vi "input_channel_tester_v2.vi"(10 "Refnums of Controls":T1[](array[typedef])) -> ()   [LabVIEW 2017]
uses:
  <vilib>/gmath/NI_Gmath.lvlib
  <vilib>/Analysis/NI_AALBase.lvlib
  <vilib>/DAQmx/read.llb/DAQmx Read (Analog 1D Wfm NChan NSamp).vi
  <vilib>/Analysis/baseanly.llb/Mean (DBL).vi
  <vilib>/Waveform/WDTOps.llb/WDT Get Waveform Time Array DBL.vi
  <vilib>/DAQmx/configure/timing.llb/DAQmx Timing (Sample Clock).vi
  analog_data.ctl
  Utility Sub VIs/pressure_temp_mixture.ctl
  Utility Sub VIs/pulse_generator_data.ctl
  Utility Sub VIs/pulse_generator_data_charts.ctl
  refnum_array_cluster.ctl
  Utility Sub VIs/diode_charts.ctl
panel:
  in  "Diode ChartsRefnum":refnum<vi>
  in  "PG Charts Refnum":refnum<vi>
  in  "Measurements Data Refnum":refnum<vi>
  in  "Pressure/Temperature/Mixture Properties Refnum":refnum<vi>
  out "Array":T2[](array[typedef])
  out "error out":errorcluster
  in  "stop":bool
  # "Test Section"
  # "Pulse Gen"
  # "Saturation\nPressure [Pa]"
  # "Saturation\nTemperature [C]"
  # "Pressure [Pa]"
  # "Temperature [C]"
  # "Liquid Tank"
  # "Separator"
  # "Liquid Inlet"
  # "Vapor Tank"
  # "Vapor Inlet"
  # "Test Section"
  # "Upper Dev Section"
  # "Lower Dev Section"
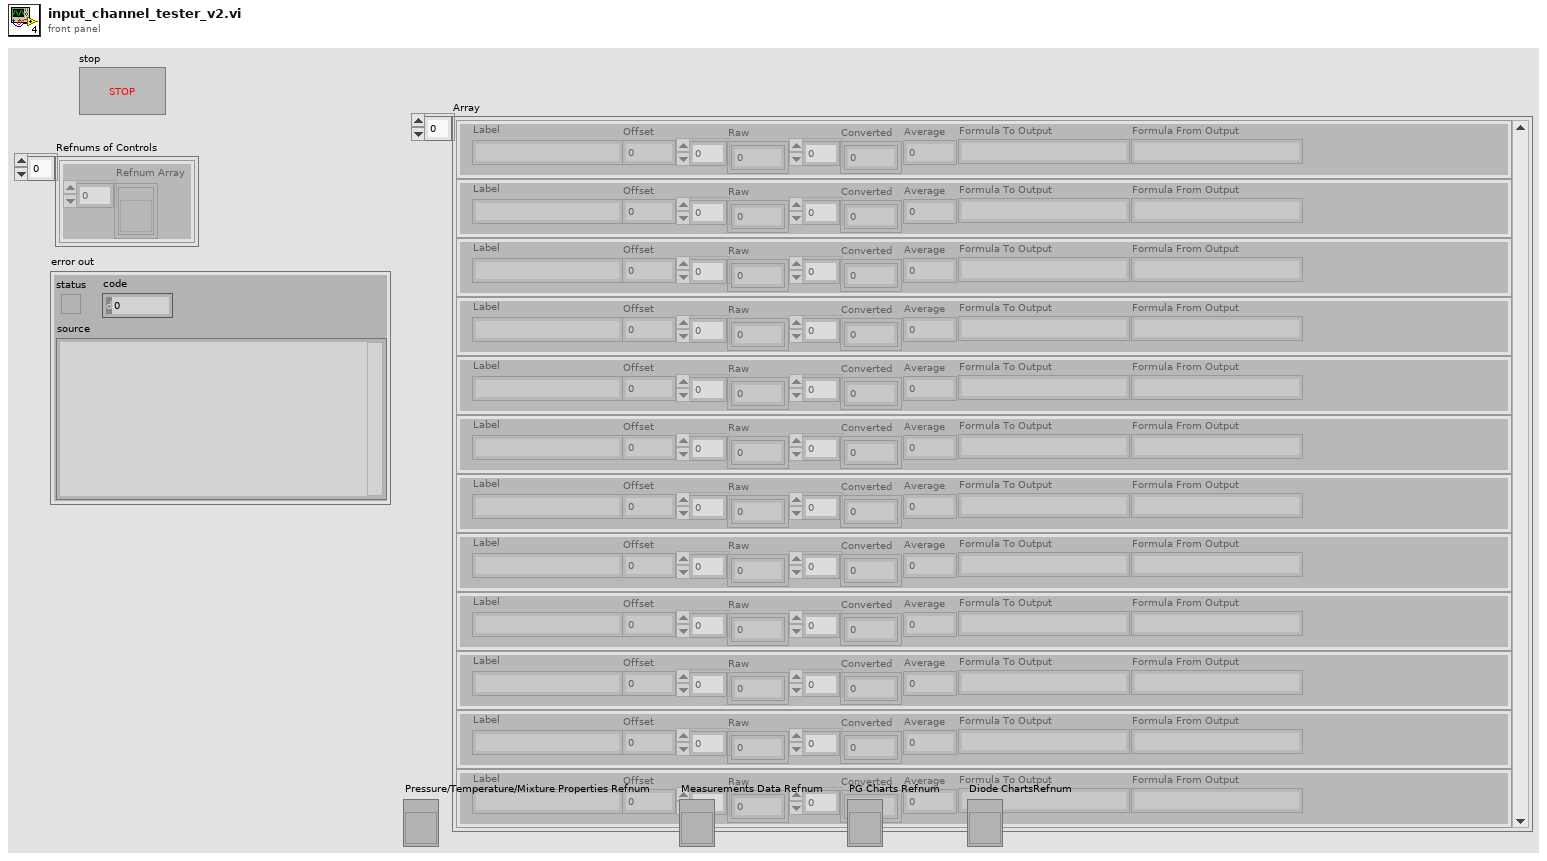
[diagram p1: front panel]
types:
  T1 = typedef "refnum_array_cluster.ctl" = cluster{"Refnum Array":refnum<vi>[]}
  T2 = typedef "analog_data.ctl" = cluster{"Label":string, "Offset":dbl, "Raw":dbl[], "Converted":dbl[], "Average":dbl, "Formula To Output":string, "Formula From Output":string}
  T3 = typedef "analog_data_channel_pkg.ctl" = cluster{"Analog Input Channel":T4, "Analog Data":T2}
  T4 = typedef "input_channel.ctl" = cluster{"Channel Name":string, "Physical Channel":tag, "Sensor Type":enum16{"Absolute Pressure", "Gauge Pressure", "Differential Pressure", "Temperature", "Mass Flow Rate", "Density", "Other"}, "Signal Type":enum16{"Voltage", "Current", "Temperature"}, "Terminal Configuration":i32, "Minimum Value":dbl, "Maximum Value":dbl, "TC Type":i32, "Sensor Min":dbl, "Sensor Max":dbl, "Sensor Offset":dbl, "Sensor Unit":enum16{"psi", "Pa", "inH2O", "inHg", "C", "K", "g/s", "g/cm3", "Volt", "Amp", ""}, "Output Unit":enum16{"psi", "Pa", "inH2O", "inHg", "C", "K", "g/s", "g/cm3", "Volt", "Amp", ""}, "Unit Conversion":dbl, "Active":bool, "Input Type":enum16{"DAQ", "Add-On"}}
  T5 = typedef "index_array_cluster.ctl" = cluster{"Index Array":i32[]}
  T6 = typedef "pressure_temp_mixture.ctl" = cluster{"Line Densities\n[g/cm^3]":cluster{"Vapor Line":dbl, "Liquid Line":dbl}, "Mixture Properties":cluster{"Enthalpy":dbl, "Quality [-]":dbl}, "Component PTs":cluster{"Liquid Tank P":dbl, "Liquid Tank T":dbl, "Liquid Tank Sat P":dbl, "Liquid Tank Sat T":dbl, "Separator P":dbl, "Separator T":dbl, "Separator Sat P":dbl, "Separator Sat T":dbl, "Liquid Inlet P":dbl, "Liquid Inlet T":dbl, "Liquid Inlet Sat P":dbl, "Liquid Inlet Sat T":dbl, "Vapor Tank P":dbl, "Vapor Tank T":dbl, "Vapor Tank Sat P":dbl, "Vapor Tank Sat T":dbl, "Vapor Inlet P":dbl, "Vapor Inlet T":dbl, "Vapor Inlet Sat P":dbl, "Vapor Inlet Sat T":dbl, "Test Section P":dbl, "Test Section T":dbl, "Test Section Sat P":dbl, "Test Section Sat T":dbl, "Upper Dev Section P":dbl, "Upper Dev Section T":dbl, "Upper Dev Section Sat P":dbl, "Upper Dev Section Sat T":dbl, "Lower Dev Section P":dbl, "Lower Dev Section T":dbl, "Lower Dev Section Sat P":dbl, "Lower Dev Section Sat T":dbl}, "Ambient Pressure [Pa]":dbl, "Mixing Tee":cluster{"Venturi dP":dbl, "PGminiPressure":dbl, "PGminiTemperature":dbl}}
  T7 = cluster{"[0]":dbl, "[1]":dbl, "[2]":dbl, "[3]":dbl, "[4]":dbl, "[5]":dbl, "[6]":dbl, "[7]":dbl, "[8]":dbl, "[9]":dbl, "[10]":dbl, "[11]":dbl, "[12]":dbl, "[13]":dbl, "[14]":dbl, "[15]":dbl, "[16]":dbl, "[17]":dbl, "[18]":dbl, "[19]":dbl, "[20]":dbl, "[21]":dbl, "[22]":dbl, "[23]":dbl, "[24]":dbl, "[25]":dbl, "[26]":dbl, "[27]":dbl, "[28]":dbl, "[29]":dbl, "[30]":dbl, "[31]":dbl}
  T8 = cluster{"Mass Flow Rate [g/s]":dbl, "Mass Flow Rate [g/s]":dbl}
  T9 = cluster{"[0]":dbl, "[1]":dbl, "[2]":dbl, "[3]":dbl, "[4]":dbl, "[5]":dbl, "[6]":dbl, "[7]":dbl, "[8]":dbl, "[9]":dbl, "[10]":dbl, "[11]":dbl, "[12]":dbl, "[13]":dbl, "[14]":dbl, "[15]":dbl}
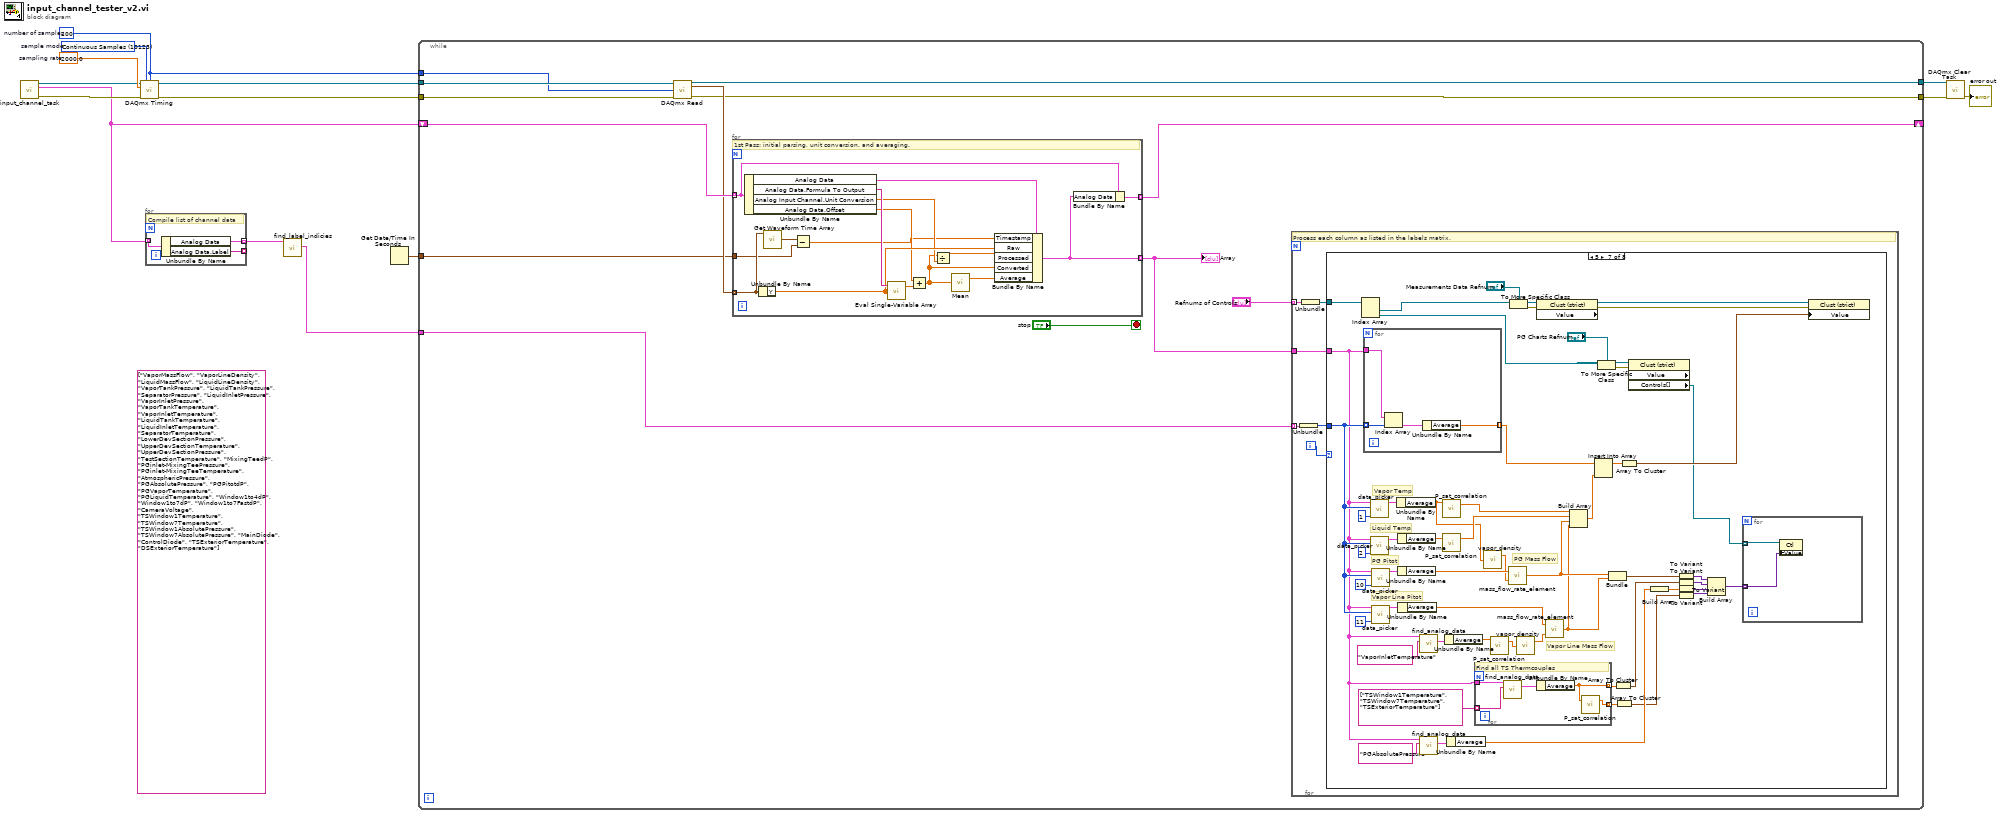
[diagram p0: block diagram]
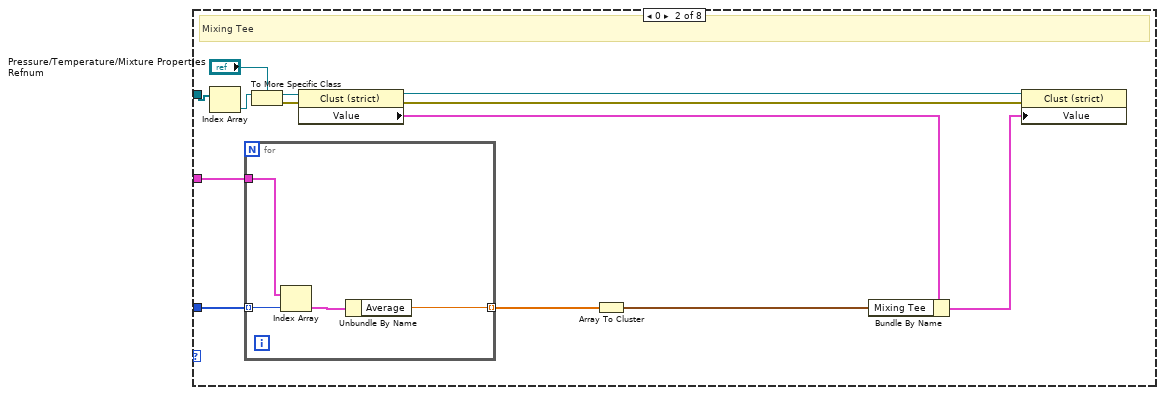
[diagram p3: hidden frame]
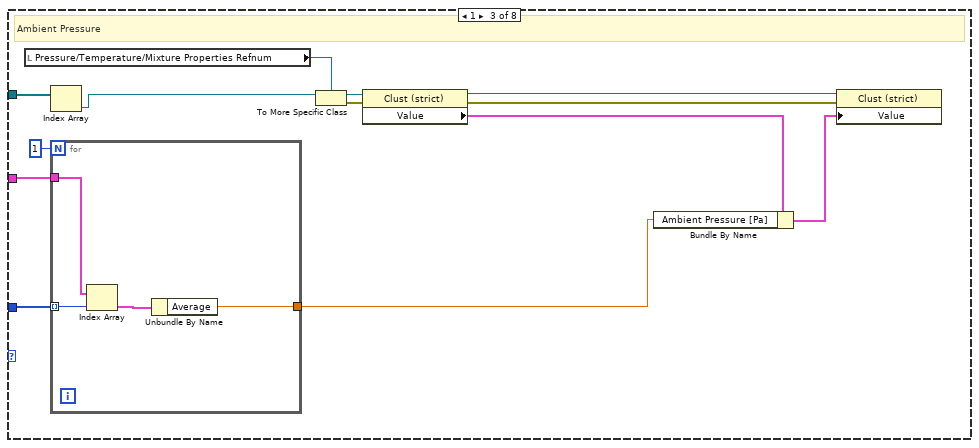
[diagram p4: hidden frame]
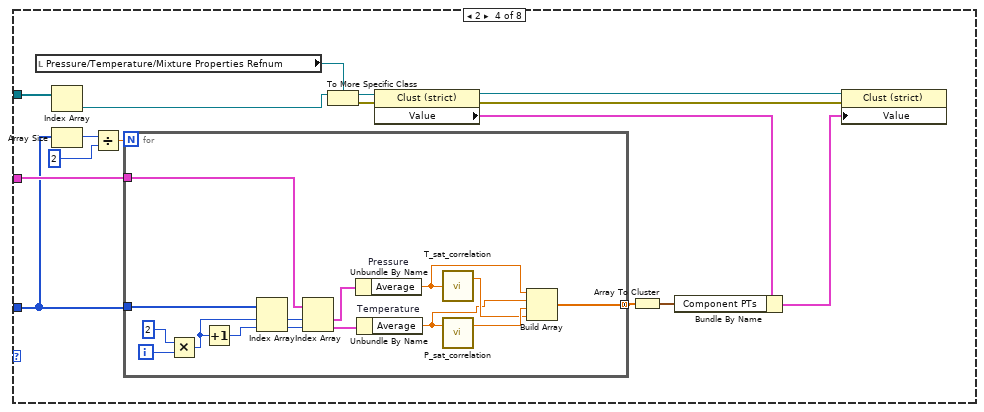
[diagram p5: hidden frame]
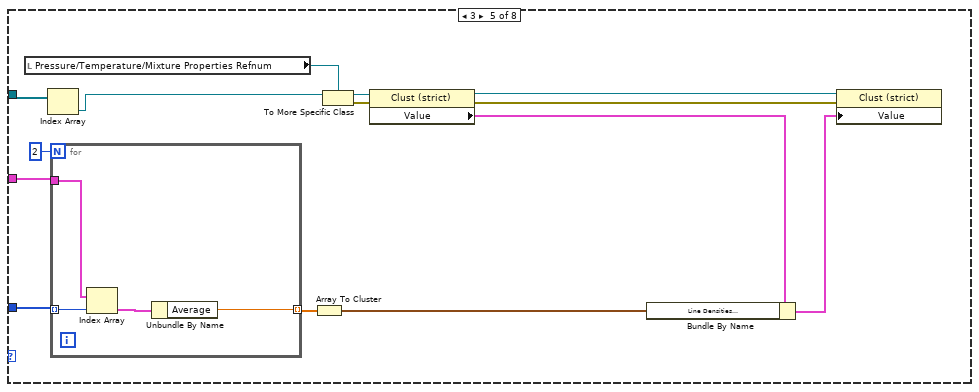
[diagram p6: hidden frame]
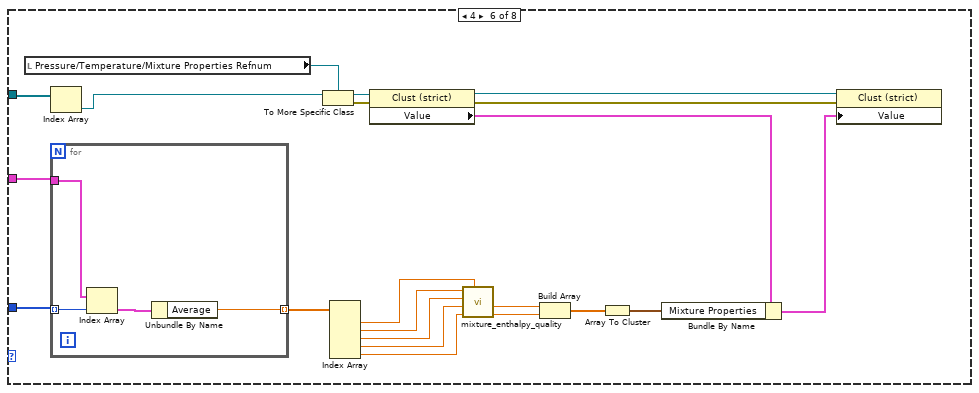
[diagram p7: hidden frame]
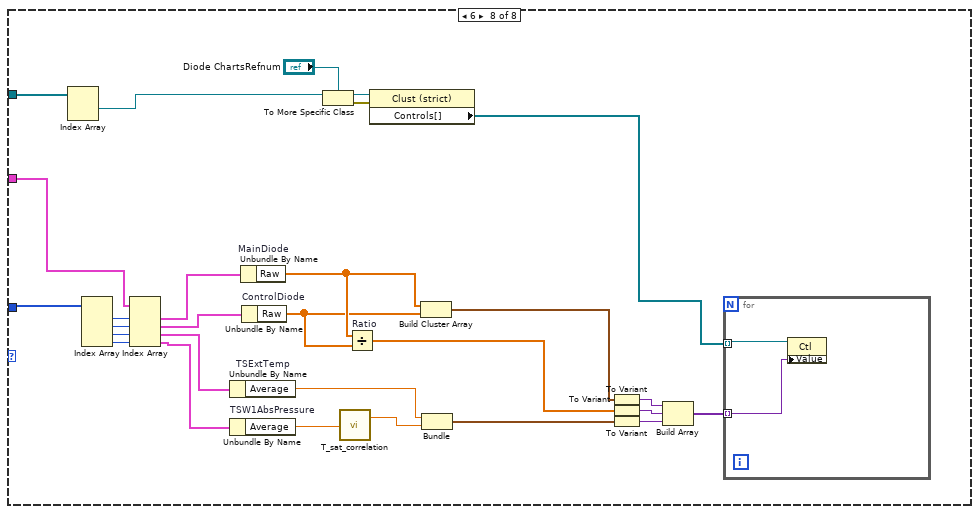
[diagram p8: hidden frame]
diagram:
  (unwired) string[] ["VaporMassFlow", "VaporLineDensity", "LiquidMassFlow", "LiquidLineDensity", "VaporTankPressure", "LiquidTankPressure", "SeparatorPressure", "LiquidInletPressure", "VaporInletPressure", "VaporTankTemperature", "VaporInletTemperature", "LiquidTankTemperature", "LiquidInletTemperature", "SeparatorTemperature", "LowerDevSectionPressure", "UpperDevSectionTemperature", "UpperDevSectionPressure", "TestSectionTemperature", "MixingTeedP", "PGinlet-MixingTeePressure", "PGinlet-MixingTeeTemperature", "AtmosphericPressure", "PGAbsolutePressure", "PGPitotdP", "PGVaporTemperature", "PGLiquidTemperature", "Window1to4dP", "Window1to7dP", "Window1to7FastdP", "CameraVoltage", "TSWindow1Temperature", "TSWindow7Temperature", "TSWindow1AbsolutePressure", "TSWindow7AbsolutePressure", "MainDiode", "ControlDiode", "TSExteriorTemperature", "DSExteriorTemperature"] ("Array 2")
  w14 = 10123 items=["Finite Samples"=10178, "Continuous Samples"=10123, "Hardware Timed Single Point"=12522]  # sample mode
  w13 = 2000.0  # sampling rate
  w4 = 200  # number of samples
  n1 = call "input_channel_task.vi"() -> ("error out"=w11:errorcluster, "Active Analog Channel-Data Packages"=w3:T3[], "task out"=w12:refnum<k21>)  [unwired: 9 in]
  n2 = call-poly <vilib>:"DAQmx Timing.vi"("task/channels in"=w12, "sample mode"=w14, "samples per channel"=w4, "rate"=w13, "error in"=w11) -> ("task out"=w10:refnum<k21>, "error out"=w9:errorcluster)  [unwired: 9 in]
  n3 = for {
    tunnel: w3 -> [w17] mode=indexing
    tunnel: [w16] -> w2 mode=indexing
    tunnel: [w15] -> _ mode=indexing
    # "Compile list of channel data"
    n4 = Unbundle By Name(w17) -> ("Analog Data"=w16:T2, "Analog Data.Label"=w15:string)
  }
  n5 = call "find_label_indicies.vi"("haystack"=w2) -> ("Indicies"=w1:T5[])  [unwired: 8 in, 2 out]
  n6 = Get Date/Time In Seconds() -> (seconds since 1Jan1904=w5:timestamp)
  n7 = while {
    tunnel: w10 -> [w28]
    tunnel: w9 -> [w27]
    tunnel: [w25] -> w7
    tunnel: [w24] -> w8
    tunnel: w5 -> [w23]
    tunnel: w4 -> [w22]
    tunnel: w1 -> [w19]
    shift-right: [w20] -> _
    shift-left: w3 -> [w29]
    stop <- "stop" stop-if-true
    n8 = call-poly <vilib>:"DAQmx Read.vi"("task/channels in"=w28, "number of samples per channel"=w22, "error in"=w27) -> ("task out"=w24:refnum<k21>, "data"=w26:waveform(dbl)[], "error out"=w25:errorcluster)  [unwired: 10 in]
    n9 = for {
      tunnel: w29 -> [w243] mode=indexing
      tunnel: w26 -> [w255] mode=indexing
      tunnel: [w242] -> w21 mode=indexing
      tunnel: w23 -> [w245]
      tunnel: [w241] -> w20 mode=indexing
      # "1st Pass: initial parsing, unit conversion, and averaging."
      n10 = Unbundle By Name(w243) -> ("Analog Data"=w256:T2, "Analog Data.Formula To Output"=w254:string, "Analog Input Channel.Unit Conversion"=w251:dbl, "Analog Data.Offset"=w247:dbl)
      n11 = Unbundle By Name(w255) -> ("Y"=w253:dbl[])
      n12 = call-poly <vilib>:"Get Waveform Time Array.vi"("waveform in"=w255) -> ("X array"=w246:timestamp[])  [unwired: 9 in, 1 out]
      n13 = Subtract(x=w246, y=w245) -> (x-y=w244:dbl[])
      n14 = call <vilib>:"Eval Single-Variable Array.vi"("X Values"=w253, "formula"=w254) -> ("Y Values"=w249:dbl[])  [unwired: 1 in, 1 out]
      n15 = Add(x=w247, y=w249) -> (x+y=w248:dbl[])
      n16 = Divide(x=w248, y=w251) -> (x/y=w250:dbl[])
      n17 = call-poly <vilib>:"Mean.vi"("X"=w248) -> ("mean"=w252:dbl)  [unwired: 1 out]
      n18 = Bundle By Name(cluster=w256, "Timestamp"=w244, "Raw"=w253, "Processed"=w250, "Converted"=w248, "Average"=w252) -> (w242:T2)
      n19 = Bundle By Name(cluster=w243, "Analog Data"=w242) -> (w241:T3)
    }
    "Array" <- w21
    n20 = for {
      tunnel: w21 -> [w35]
      tunnel: w19 -> [w32] mode=indexing
      tunnel: "Refnums of Controls" -> [w34] mode=indexing
      i -> [w36]
      # "Process each column as listed in the labels matrix."
      n21 = Unbundle(w32) -> ("Index Array"=w31:i32[])
      n22 = Unbundle(w34) -> ("Refnum Array"=w33:refnum<vi>[])
      n23 = case shown="5" w36 {
        tunnel: w31 -> [_ w42 w59 w78 w107 w132 w186 w228]
        tunnel: w33 -> [_ w38 w55 w72 w103 w121 w156 w234]
        tunnel: w35 -> [_ w41 w60 w79 w108 w133 w161 w226]
        frame Default {
        }
        frame 0 {
          # "Mixing Tee"
          n24 = Index Array(array=w38) -> (element=w37:refnum<vi>)  [unwired: 1 in]
          n25 = for {
            tunnel: w42 -> [w53] mode=indexing
            tunnel: w41 -> [w52]
            tunnel: [w50] -> w40 mode=indexing
            n26 = Index Array(array=w52, index=w53) -> (element=w51:T2)
            n27 = Unbundle By Name(w51) -> ("Average"=w50:dbl)
          }
          n28 = To More Specific Class(target class="Pressure/Temperature/Mixture Properties Refnum", reference=w37) -> (specific class reference=w48:refnum<vi>, error out=w47:errorcluster)  [unwired: 1 in]
          n29 = property class="Clust (strict)"(reference=w48, error in=w47) -> (reference out=w43:refnum<vi>, error out=w44:errorcluster, "Value"=w46:T6)
          n30 = Array To Cluster(array=w40) -> (cluster=w39:cluster{"[0]":dbl, "[1]":dbl, "[2]":dbl})
          n31 = Bundle By Name(cluster=w46, "Mixing Tee"=w39) -> (w45:T6)
          n32 = property class="Clust (strict)"(reference=w43, error in=w44, "Value"=w45) -> ()  [unwired: 2 out]
        }
        frame 1 {
          # "Ambient Pressure"
          n33 = local read "Pressure/Temperature/Mixture Properties Refnum"() -> (w57:refnum<vi>)
          n34 = Index Array(array=w55) -> (element=w54:refnum<vi>)  [unwired: 1 in]
          n35 = for {
            N: 1 -> [_]
            tunnel: w59 -> [w70] mode=indexing
            tunnel: w60 -> [w69]
            tunnel: [w67] -> w58
            n36 = Index Array(array=w69, index=w70) -> (element=w68:T2)
            n37 = Unbundle By Name(w68) -> ("Average"=w67:dbl)
          }
          n38 = To More Specific Class(target class=w57, reference=w54) -> (specific class reference=w66:refnum<vi>, error out=w65:errorcluster)  [unwired: 1 in]
          n39 = property class="Clust (strict)"(reference=w66, error in=w65) -> (reference out=w61:refnum<vi>, error out=w62:errorcluster, "Value"=w64:T6)
          n40 = Bundle By Name(cluster=w64, "Ambient Pressure [Pa]"=w58) -> (w63:T6)
          n41 = property class="Clust (strict)"(reference=w61, error in=w62, "Value"=w63) -> ()  [unwired: 2 out]
        }
        frame 2 {
          n42 = local read "Pressure/Temperature/Mixture Properties Refnum"() -> (w80:refnum<vi>)
          n43 = Index Array(array=w72) -> (element=w71:refnum<vi>)  [unwired: 1 in]
          n44 = Array Size(array=w78) -> (size(s)=w76:i32)
          n45 = Divide(x=w76, y=2) -> (x/y=w77:dbl)
          n46 = for {
            N: w77 -> [_]
            tunnel: w78 -> [w97]
            tunnel: w79 -> [w101]
            tunnel: [w87] -> w74 mode=concatenating
            i -> [w99]
            n47 = Multiply(x=2, y=w99) -> (x*y=w95:i32)
            n48 = Increment(x=w95) -> (x+1=w96:i32)
            n49 = Index Array(array=w97, index #1=w95, index #2=w96) -> (element #1=w94:i32, element #2=w93:i32)
            n50 = Index Array(array=w101, index #1=w94, index #2=w93) -> (element #1=w100:T2, element #2=w92:T2)
            n51 = Unbundle By Name "Pressure"(w100) -> ("Average"=w89:dbl)
            n52 = Unbundle By Name "Temperature"(w92) -> ("Average"=w88:dbl)
            n53 = call "T_sat_correlation.vi"("P [Pa]"=w89) -> ("T Sat [C]"=w90:dbl)  [unwired: 1 out]
            n54 = call "P_sat_correlation.vi"("Temperature[C]"=w88) -> ("P Sat[Pa]"=w91:dbl)  [unwired: 1 in, 1 out]
            n55 = Build Array(w89, w88, w91, w90) -> (w87:dbl[])
          }
          n56 = To More Specific Class(target class=w80, reference=w71) -> (specific class reference=w86:refnum<vi>, error out=w85:errorcluster)  [unwired: 1 in]
          n57 = property class="Clust (strict)"(reference=w86, error in=w85) -> (reference out=w81:refnum<vi>, error out=w82:errorcluster, "Value"=w84:T6)
          n58 = Array To Cluster(array=w74) -> (cluster=w73:T7)
          n59 = Bundle By Name(cluster=w84, "Component PTs"=w73) -> (w83:T6)
          n60 = property class="Clust (strict)"(reference=w81, error in=w82, "Value"=w83) -> ()  [unwired: 2 out]
        }
        frame 3 {
          n61 = local read "Pressure/Temperature/Mixture Properties Refnum"() -> (w109:refnum<vi>)
          n62 = Index Array(array=w103) -> (element=w102:refnum<vi>)  [unwired: 1 in]
          n63 = for {
            N: 2 -> [_]
            tunnel: w107 -> [w119] mode=indexing
            tunnel: w108 -> [w118]
            tunnel: [w116] -> w106 mode=indexing
            n64 = Index Array(array=w118, index=w119) -> (element=w117:T2)
            n65 = Unbundle By Name(w117) -> ("Average"=w116:dbl)
          }
          n66 = Array To Cluster(array=w106) -> (cluster=w105:cluster{"[0]":dbl, "[1]":dbl})
          n67 = To More Specific Class(target class=w109, reference=w102) -> (specific class reference=w115:refnum<vi>, error out=w114:errorcluster)  [unwired: 1 in]
          n68 = property class="Clust (strict)"(reference=w115, error in=w114) -> (reference out=w110:refnum<vi>, error out=w111:errorcluster, "Value"=w113:T6)
          n69 = Bundle By Name(cluster=w113, "Line Densities\n[g/cm^3]"=w105) -> (w112:T6)
          n70 = property class="Clust (strict)"(reference=w110, error in=w111, "Value"=w112) -> ()  [unwired: 2 out]
        }
        frame 4 {
          n71 = local read "Pressure/Temperature/Mixture Properties Refnum"() -> (w134:refnum<vi>)
          n72 = Index Array(array=w121) -> (element=w120:refnum<vi>)  [unwired: 1 in]
          n73 = for {
            tunnel: w132 -> [w144] mode=indexing
            tunnel: w133 -> [w143]
            tunnel: [w141] -> w131 mode=indexing
            n74 = Index Array(array=w143, index=w144) -> (element=w142:T2)
            n75 = Unbundle By Name(w142) -> ("Average"=w141:dbl)
          }
          n76 = To More Specific Class(target class=w134, reference=w120) -> (specific class reference=w140:refnum<vi>, error out=w139:errorcluster)  [unwired: 1 in]
          n77 = Index Array(array=w131) -> (element #1=w126:dbl, element #2=w125:dbl, element #3=w124:dbl, element #4=w123:dbl, element #5=w122:dbl)  [unwired: 5 in]
          n78 = property class="Clust (strict)"(reference=w140, error in=w139) -> (reference out=w135:refnum<vi>, error out=w136:errorcluster, "Value"=w138:T6)
          n79 = call "mixture_enthalpy_quality.vi"("Vapor Inlet Pressure [Pa]"=w126, "Separator Temp [C]"=w122, "Liquid Inlet Temp [C]"=w123, "Vapor Flow Rate [g/s]"=w124, "Liquid Flow Rate [g/s]"=w125) -> ("Quality [-]"=w129:dbl, "mixture enthalpy"=w130:dbl)  [unwired: 2 out]
          n80 = Build Array(w130, w129) -> (w128:dbl[])
          n81 = Array To Cluster(array=w128) -> (cluster=w127:cluster{"[0]":dbl, "[1]":dbl})
          n82 = Bundle By Name(cluster=w138, "Mixture Properties"=w127) -> (w137:T6)
          n83 = property class="Clust (strict)"(reference=w135, error in=w136, "Value"=w137) -> ()  [unwired: 2 out]
        }
        frame 5 {
          # "Vapor Line Mass Flow"
          # "PG Mass Flow"
          # "PG Pitot"
          # "Vapor Line Pitot"
          # "Liquid Temp"
          # "Vapor Temp"
          n84 = Index Array(array=w156) -> (element #1=w158:refnum<vi>, element #2=w157:refnum<vi>)  [unwired: 2 in]
          n85 = for {
            tunnel: w186 -> [w210] mode=indexing
            tunnel: w161 -> [w209]
            tunnel: [w207] -> w177 mode=indexing
            n86 = Index Array(array=w209, index=w210) -> (element=w208:T2)
            n87 = Unbundle By Name(w208) -> ("Average"=w207:dbl)
          }
          n88 = call "data_picker.vi"("index"=1, "Indicies"=w186, "Data in"=w161) -> ("Data Out"=w168:T2)  [unwired: 8 in]
          n89 = call "data_picker.vi"("index"=2, "Indicies"=w186, "Data in"=w161) -> ("Data Out"=w192:T2)  [unwired: 8 in]
          n90 = call "data_picker.vi"("index"=10, "Indicies"=w186, "Data in"=w161) -> ("Data Out"=w189:T2)  [unwired: 8 in]
          n91 = call "data_picker.vi"("index"=11, "Indicies"=w186, "Data in"=w161) -> ("Data Out"=w190:T2)  [unwired: 8 in]
          n92 = Unbundle By Name(w168) -> ("Average"=w145:dbl)
          n93 = Unbundle By Name(w192) -> ("Average"=w191:dbl)
          n94 = Unbundle By Name(w189) -> ("Average"=w185:dbl)
          n95 = Unbundle By Name(w190) -> ("Average"=w178:dbl)
          n96 = call "find_analog_data.vi"("Needle"="VaporInletTemperature", "Haystack"=w161) -> ("Needle Out"=w182:T2)  [unwired: 7 in, 2 out]
          n97 = call "find_analog_data.vi"("Needle"="PGAbsolutePressure", "Haystack"=w161) -> ("Needle Out"=w166:T2)  [unwired: 7 in, 2 out]
          n98 = call "P_sat_correlation.vi"("Temperature[C]"=w145) -> ("P Sat[Pa]"=w176:dbl)  [unwired: 1 in, 1 out]
          n99 = call "P_sat_correlation.vi"("Temperature[C]"=w191) -> ("P Sat[Pa]"=w175:dbl)  [unwired: 1 in, 1 out]
          n100 = Unbundle By Name(w182) -> ("Average"=w181:dbl)
          n101 = Unbundle By Name(w166) -> ("Average"=w165:dbl)
          n102 = for {
            tunnel: string[] ["TSWindow1Temperature", "TSWindow7Temperature", "TSExteriorTemperature"] ("Needle") -> [w205] mode=indexing
            tunnel: w161 -> [w206]
            tunnel: [w203] -> w160 mode=indexing
            tunnel: [w202] -> w159 mode=indexing
            # "Find all TS Thermcouples"
            n103 = call "find_analog_data.vi"("Needle"=w205, "Haystack"=w206) -> ("Needle Out"=w204:T2)  [unwired: 7 in, 2 out]
            n104 = Unbundle By Name(w204) -> ("Average"=w203:dbl)
            n105 = call "P_sat_correlation.vi"("Temperature[C]"=w203) -> ("P Sat[Pa]"=w202:dbl)  [unwired: 1 in, 1 out]
          }
          n106 = call "vapor_density.vi"("Vapor Temp [C]"=w145) -> ("Vapor Density[g/cm3]"=w184:dbl)  [unwired: 1 out]
          n107 = call "P_sat_correlation.vi"("Temperature[C]"=w181) -> ("P Sat[Pa]"=w180:dbl)  [unwired: 1 in, 1 out]
          n108 = call "mass_flow_rate_element.vi"("Density [g/cm3]"=w184, "dP [Pa]"=w185) -> ("Mass Flow Rate [g/s]"=w164:dbl)
          n109 = To More Specific Class(target class="Measurements Data Refnum", reference=w158) -> (specific class reference=w199:refnum<vi>, error out=w198:errorcluster)  [unwired: 1 in]
          n110 = call "vapor_density.vi"("Vapor Temp [C]"=w180) -> ("Vapor Density[g/cm3]"=w179:dbl)  [unwired: 1 out]
          n111 = property class="Clust (strict)" props=["Value"](reference=w199, error in=w198) -> (reference out=w196:refnum<vi>, error out=w197:errorcluster)  [unwired: 1 out]
          n112 = call "mass_flow_rate_element.vi"("Density [g/cm3]"=w179, "dP [Pa]"=w178) -> ("Mass Flow Rate [g/s]"=w163:dbl)
          n113 = Build Array(w176, w175, w164, w163) -> (w174:dbl[])
          n114 = Insert Into Array(array=w177, new element=w174) -> (w173:dbl[])  [unwired: 1 in]
          n115 = To More Specific Class(target class="PG Charts Refnum", reference=w157) -> (specific class reference=w171:refnum<vi>, error out=w170:errorcluster)  [unwired: 1 in]
          n116 = Bundle("Mass Flow Rate [g/s]"=w164, "Mass Flow Rate [g/s]"=w163) -> (w154:T8)  [unwired: 1 in]
          n117 = Array To Cluster(array=w160) -> (cluster=w153:cluster{"[0]":dbl, "[1]":dbl, "[2]":dbl})
          n118 = Array To Cluster(array=w159) -> (cluster=w151:cluster{"[0]":dbl, "[1]":dbl})
          n119 = Array To Cluster(array=w173) -> (cluster=w172:T9)
          n120 = property class="Clust (strict)" props=["Value", "Controls[]"](reference=w171, error in=w170) -> ("Controls[]"=w155:refnum<vi>[])  [unwired: 3 out]
          n121 = Build Array(w165) -> (w152:dbl[])
          n122 = To Variant(anything=w154) -> (Variant=w150:variant)
          n123 = To Variant(anything=w153) -> (Variant=w149:variant)
          n124 = To Variant(anything=w152) -> (Variant=w148:variant)
          n125 = To Variant(anything=w151) -> (Variant=w147:variant)
          n126 = Build Array(w150, w149, w148, w147) -> (w146:variant[])
          n127 = for {
            tunnel: w155 -> [w201] mode=indexing
            tunnel: w146 -> [w200] mode=indexing
            n128 = property class="Ctl"(reference=w201, "Value"=w200) -> ()  [unwired: 1 in, 2 out]
          }
          n129 = property class="Clust (strict)"(reference=w196, error in=w197, "Value"=w172) -> ()  [unwired: 2 out]
        }
        frame 6 {
          n130 = Index Array(array=w234) -> (element #1=w235:refnum<vi>)  [unwired: 2 in, 1 out]
          n131 = Index Array(array=w228) -> (element #1=w223:i32, element #2=w227:i32, element #3=w225:i32, element #4=w224:i32)  [unwired: 4 in]
          n132 = Index Array(array=w226, index #1=w223, index #2=w227, index #3=w225, index #4=w224) -> (element #1=w222:T2, element #2=w221:T2, element #3=w216:T2, element #4=w215:T2)
          n133 = Unbundle By Name "TSExtTemp"(w216) -> ("Average"=w213:dbl)
          n134 = Unbundle By Name "TSW1AbsPressure"(w215) -> ("Average"=w214:dbl)
          n135 = Unbundle By Name "MainDiode"(w222) -> ("Raw"=w220:dbl[])
          n136 = Unbundle By Name "ControlDiode"(w221) -> ("Raw"=w219:dbl[])
          n137 = To More Specific Class(target class="Diode ChartsRefnum", reference=w235) -> (specific class reference=w238:refnum<vi>, error out=w237:errorcluster)  [unwired: 1 in]
          n138 = call "T_sat_correlation.vi"("P [Pa]"=w214) -> ("T Sat [C]"=w212:dbl)  [unwired: 1 out]
          n139 = Divide "Ratio"(x=w220, y=w219) -> (x/y=w217:dbl[])
          n140 = property class="Clust (strict)"(reference=w238, error in=w237) -> ("Controls[]"=w229:refnum<vi>[])  [unwired: 2 out]
          n141 = Build Cluster Array(w220, w219) -> (w218:cluster{dbl, dbl}[])
          n142 = Bundle("Average"=w213, "T Sat [C]"=w212) -> (w211:cluster{"Average":dbl, "T Sat [C]":dbl})  [unwired: 1 in]
          n143 = To Variant(anything=w218) -> (Variant=w233:variant)
          n144 = To Variant(anything=w217) -> (Variant=w232:variant)
          n145 = To Variant(anything=w211) -> (Variant=w231:variant)
          n146 = Build Array(w233, w232, w231) -> (w230:variant[])
          n147 = for {
            tunnel: w229 -> [w240] mode=indexing
            tunnel: w230 -> [w239] mode=indexing
            n148 = property class="Ctl"(reference=w240, "Value"=w239) -> ()  [unwired: 1 in, 2 out]
          }
        }
      }
    }
  }
  n149 = call <vilib>:"DAQmx Clear Task.vi"("task in"=w8, "error in"=w7) -> ("error out"=→"error out":errorcluster)  [unwired: 13 in]
